vi "CollectISEOnly.vi"() -> ()   [LabVIEW 2016]
uses:
  <vilib>/Platform/TimedLoop/XDataNode/timing_clust.ctl
  <vilib>/Platform/TimedLoop/XDataNode/nitl_modes.ctl
  <vilib>/Platform/TimedLoop/XDataNode/wakeup.ctl
  <vilib>/Utility/file.llb/Write Delimited Spreadsheet (string).vi
  <vilib>/Platform/TimedLoop/XDataNode/loadnilvce.vi
  <vilib>/Utility/file.llb/Write Delimited Spreadsheet (DBL).vi
  <vilib>/Platform/TimedLoop/XDataNode/XDataNode.xnode
  <resource>/objmgr/ni.var.rc
  <vilib>/Platform/TimedLoop/XDataNode/XDNodeRunTimeDep.lvlib
panel:
  out "pH Live":dbl format="%#_4g"
  out "String 4":string="NH4"
  out "String 3":string="NH4"
  out "DO Live":dbl format="%#_4g"
  in  "Buffer Size":i32=100
  out "Saving?":bool
  out "new file path (Not A Path if cancelled)":path
  in  "File Name:":string
  out "Headers":string[](array[string])
  out "error out":errorcluster
  out "String 6":string="Na"
  out "NH4 Live":dbl format="%#_4g"
  out "Na Live":dbl format="%#_4g"
  out "current sample":dbl format="%#_3g"
  out "Date":string="K"
  out "Time":string="K"
  out "iter number":i32
  in  "stop":bool
  out "All data":dbl[][](array[numeric]) format="%#3.4f"
  in  "error in":errorcluster
  out "String 2":string="NH4"
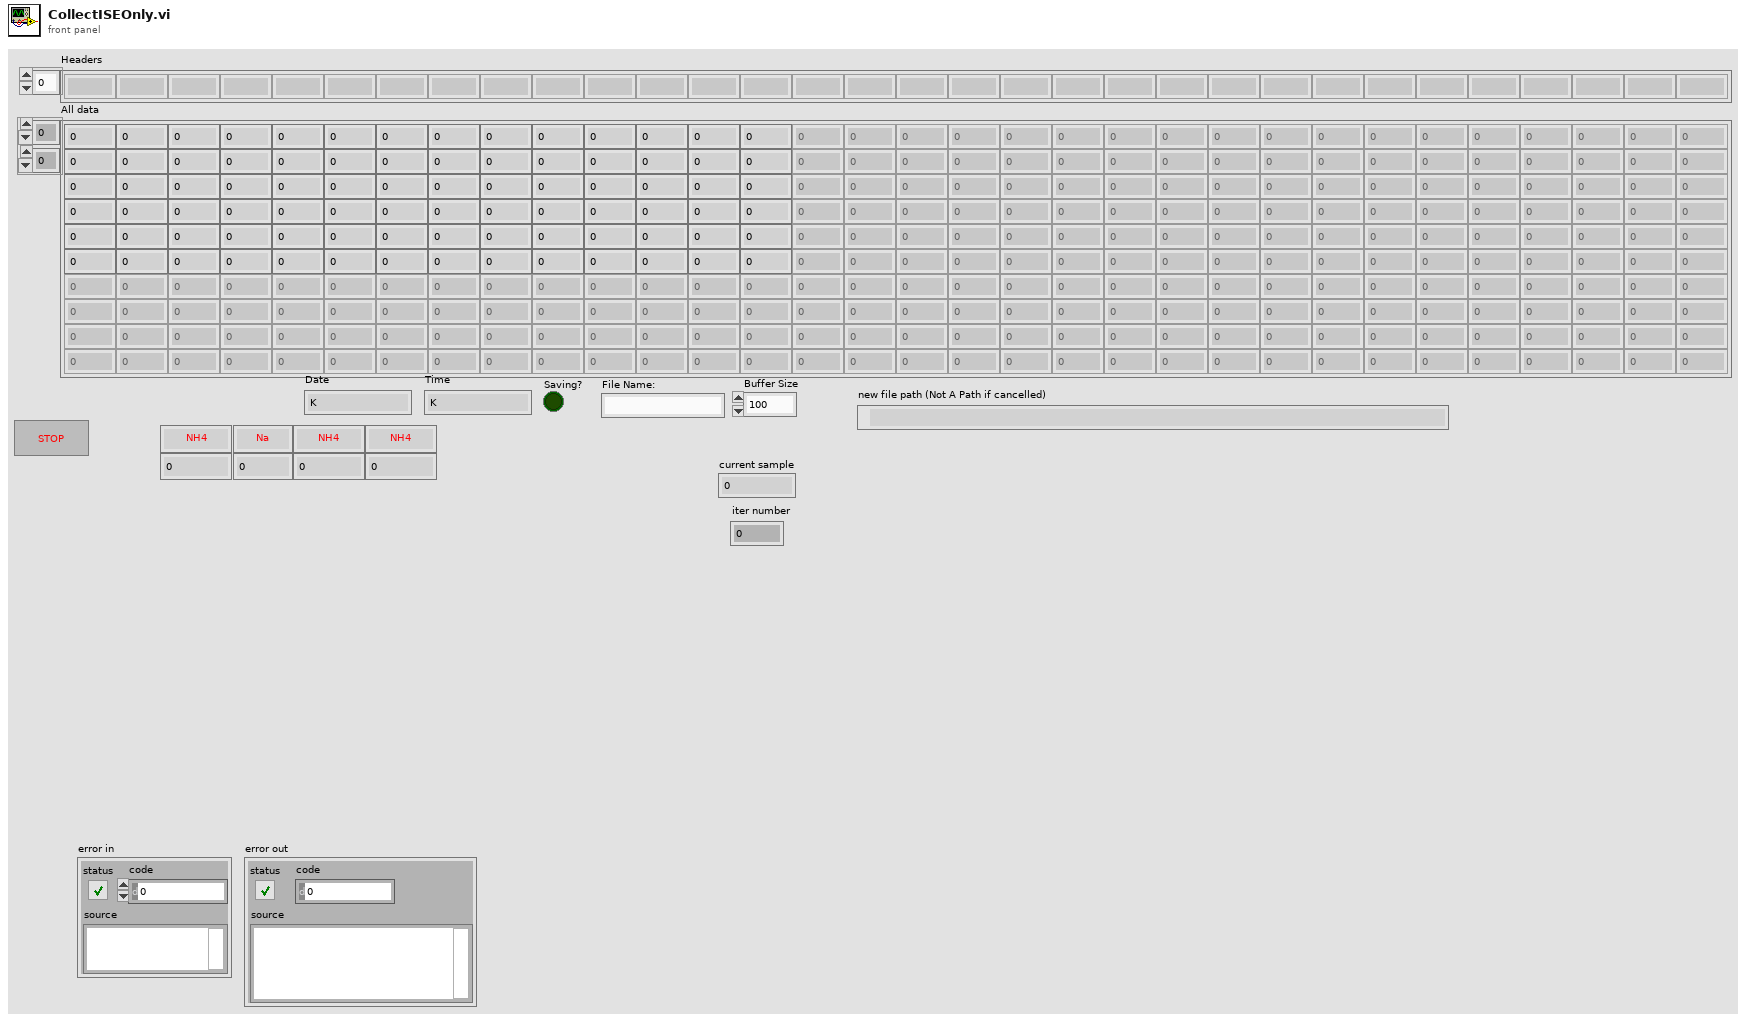
[diagram p1: front panel]
types:
  T1 = typedef "XDNodeRunTimeDep.lvlib/timing_clust.ctl" = cluster{"Expected End [f-1]":u64, "Actual End [f-1]":u64, "Finished Late? [f-1]":bool, "Expected End [i-1]":u64, "Actual End [i-1]":u64, "Finished Late? [i-1]":bool, "Expected Start [i]":u64, "Actual Start [i]":u64, "Expected Start [f]":u64, "Actual Start [f]":u64, "Source Name":string, "Structure Name":string, "Period":i64, "Deadline":i64, "Offset":i64, "Start":i64, "Priority":i32, "Timeout":i32, "Mode":T2, "Wakeup Reason":T3, "Error":errorcluster, "Source Type":string, "Secondary Source Type":string, "Global End Time":u64, "Global Start Time":u64, "Frame Duration":u64, "Iteration Duration":u64, "Assigned CPU":i32, "I/O Scan Engine Mode":u32}
  T2 = typedef "XDNodeRunTimeDep.lvlib/nitl_modes.ctl" = enum32{"No Change", "Process missed periods, maintain original phase", "Discard missed periods, maintain original phase", "Process missed periods, ignore original phase", "Discard missed periods, ignore original phase"}
  T3 = typedef "XDNodeRunTimeDep.lvlib/wakeup.ctl" = enum32{"Normal", "Aborted", "Asynchronous wakeup", "Timing source error", "Timed loop error", "Timeout"}
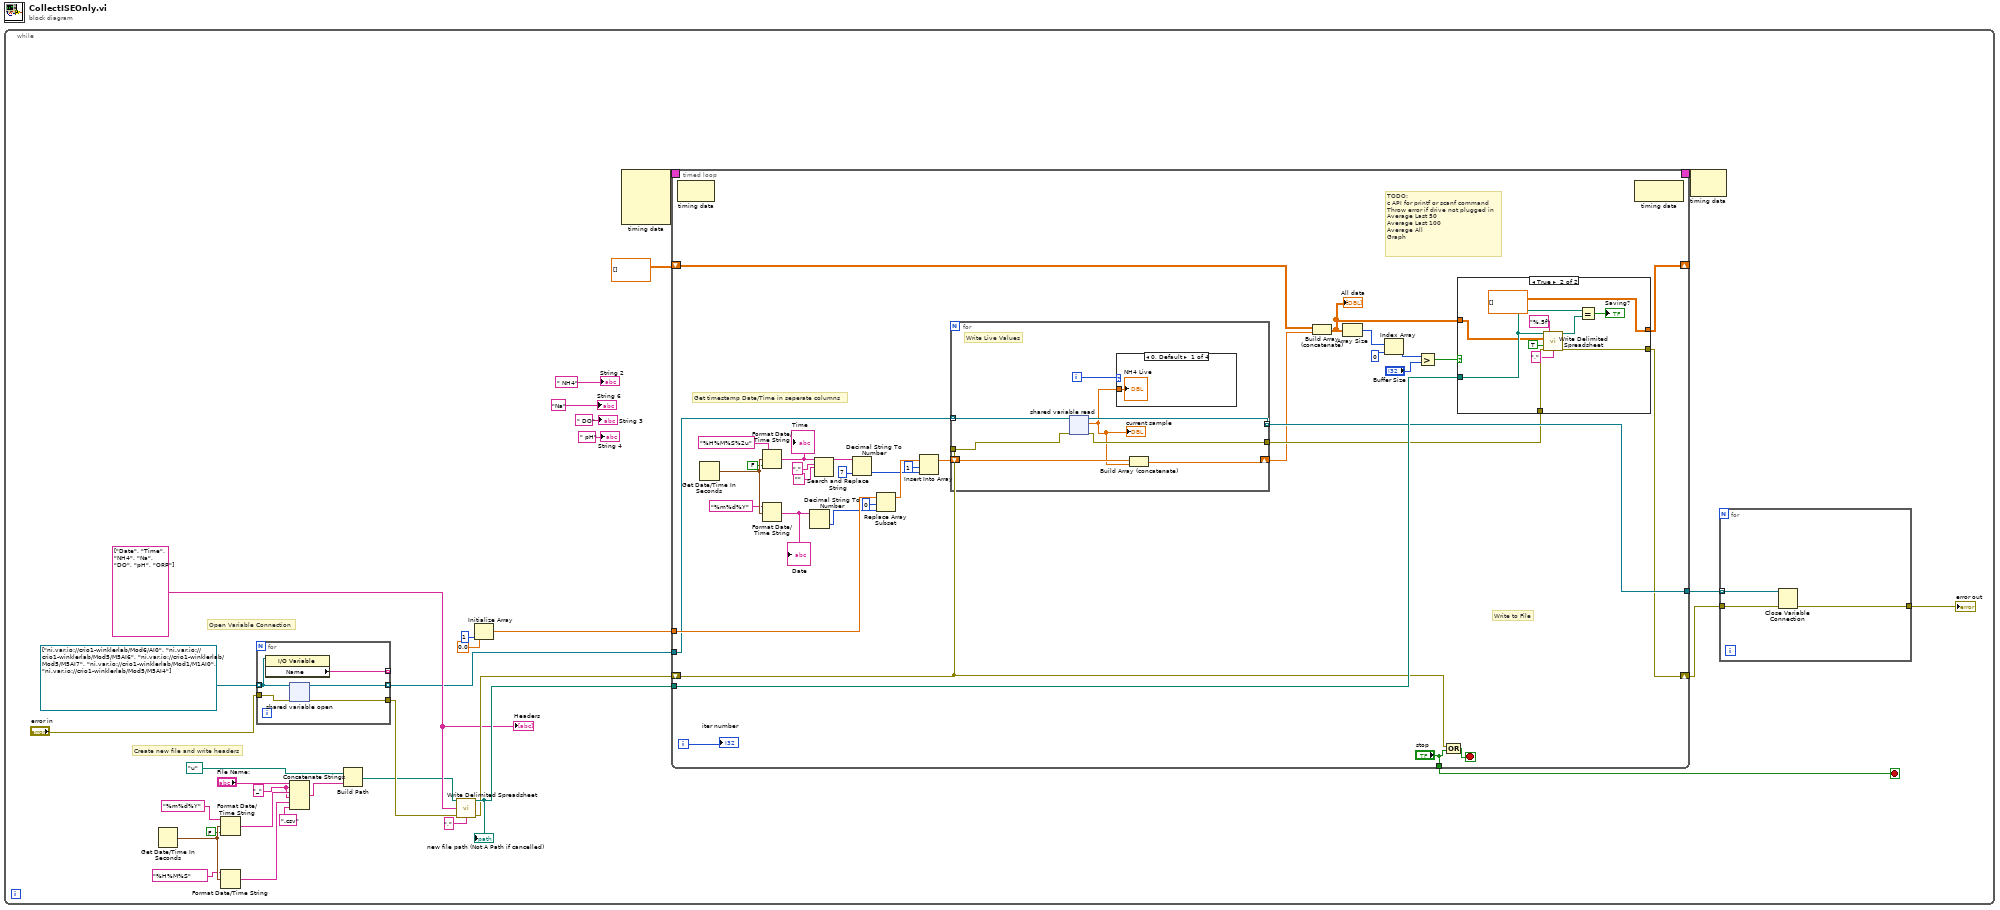
[diagram p0: block diagram]
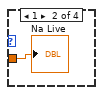
[diagram p3: hidden frame]
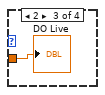
[diagram p4: hidden frame]
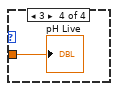
[diagram p5: hidden frame]
diagram:
  n1 = while {
    stop <- w6 stop-if-true
    w10 = "_" ("string")
    w25 = string[] ["Date", "Time", "NH4", "Na", "DO", "pH", "ORP"]
    # "Create new file and write headers"
    # "Open Variable Connection"
    n2 = Get Date/Time In Seconds() -> (seconds since 1Jan1904=w15:timestamp)
    n3 = Format Date/Time String(time format string (%c)="%m%d%Y", seconds (now)=w15, UTC format=FALSE) -> (date/time string=w11:string)
    n4 = Format Date/Time String(time format string (%c)="%H%M%S", seconds (now)=w15) -> (date/time string=w9:string)  [unwired: 1 in]
    n5 = for {
      tunnel: refnum<k21>[] ["ni.var.io://crio1-winklerlab/Mod6/AI0", "ni.var.io://crio1-winklerlab/Mod5/M5AI6", "ni.var.io://crio1-winklerlab/Mod5/M5AI7", "ni.var.io://crio1-winklerlab/Mod1/M1AI0", "ni.var.io://crio1-winklerlab/Mod5/M5AI4"] -> [w99] mode=indexing
      tunnel: "error in" -> [w102]
      tunnel: [w101] -> w22 mode=indexing
      tunnel: [w100] -> w20
      tunnel: [w98] -> _ mode=indexing
      n6 = property class="I/O Variable"(reference=w99) -> ("Name"=w98:string)  [unwired: 1 in, 2 out]
      n7 = shared-variable-open(w99, w102) -> (w101:refnum<k21>, w100:errorcluster)  [unwired: 1 in]
    }
    n8 = Concatenate Strings("File Name:", w10, w11, w10, w9, ".csv" ("string")) -> (w7:string)
    n9 = Build Path(base path=path "u:/" ("Save to:"), name or relative path=w7) -> (appended path=w19:path)
    n10 = call-poly <vilib>:"Write Delimited Spreadsheet.vi"("file path (dialog if empty)"=w19, "1D data"=w25, "error in (no error)"=w20, "delimiter (\\t)"="," ("delimiter (\\t)")) -> ("new file path (Not A Path if cancelled)"=w32:path, "error out"=w30:errorcluster)  [unwired: 10 in]
    "new file path (Not A Path if cancelled)" <- w32
    n11 = Initialize Array(0.0 ("element"), 1 ("dimension size")) -> (w33:dbl[])
    n12 = node-c288() -> (w5:T1)  [unwired: 4 in]
    n13 = timed-loop {
      tunnel: w33 -> [w60]
      tunnel: w32 -> [w46]
      shift-right: [w45] -> _
      shift-left: dbl[][] [] -> [w56]
      tunnel: w22 -> [w41]
      tunnel: [w43] -> w18
      shift-right: [w37] -> w8
      shift-left: w30 -> [w38]
      tunnel: ["stop"] -> w6
      timing: w5 -> [_]
      timing-out: [_] -> w4
      i -> [w57]
      stop <- w58 stop-if-true
      # "TODO: \nc API for printf or scanf command\nThrow error if drive not plugged in\nAverage Last 50\nAverage Last 100\nAverage All\nGraph"
      # "Write to File"
      # "Get timestamp Date/Time in seperate columns"
      n14 = node-c288() -> ()  [unwired: 1 in, 1 out]
      n15 = Get Date/Time In Seconds() -> (seconds since 1Jan1904=w68:timestamp)
      n16 = Format Date/Time String(time format string (%c)="%H%M%S%2u", seconds (now)=w68, UTC format=FALSE) -> (date/time string=w64:string)
      "Time" <- w64
      n17 = Format Date/Time String(time format string (%c)="%m%d%Y", seconds (now)=w68) -> (date/time string=w54:string)  [unwired: 1 in]
      "Date" <- w54
      n18 = Decimal String To Number(string=w54) -> (number=w53:i32)  [unwired: 2 in, 1 out]
      n19 = Search and Replace String(input string=w64, search string=".", replace string="") -> (result string=w63:string)  [unwired: 5 in, 3 out]
      n20 = Decimal String To Number(string=w63, default (0L)=7) -> (number=w52:i32)  [unwired: 1 in, 1 out]
      n21 = Replace Array Subset(array=w60, new element=w53, index=0) -> (w59:dbl[])
      n22 = Insert Into Array(array=w59, index=1, new element=w52) -> (w36:dbl[])
      n23 = for {
        tunnel: w38 -> [w91]
        shift-right: [w87] -> w40
        shift-left: w36 -> [w86]
        tunnel: [w90] -> w42
        tunnel: w41 -> [w89] mode=indexing
        tunnel: [w88] -> w43 mode=indexing
        i -> [w84]
        # "Write Live Values"
        n24 = shared-variable-read(w89, w91) -> (w88:refnum<k21>, w90:errorcluster, w85:dbl)  [unwired: 1 out]
        "current sample" <- w85
        n25 = case shown="0, Default" w84 {
          tunnel: w85 -> [w92 w93 w94 w95]
          frame 0, Default {
            "NH4 Live" <- w92
          }
          frame 1 {
            "Na Live" <- w93
          }
          frame 2 {
            "DO Live" <- w94
          }
          frame 3 {
            "pH Live" <- w95
          }
        }
        n26 = Build Array (concatenate)(w86, w85) -> (w87:dbl[])
      }
      n27 = Build Array (concatenate)(w56, w40) -> (w44:dbl[][])
      "All data" <- w44
      n28 = Array Size(array=w44) -> (size(s)=w50:i32[])
      n29 = Index Array(array=w50, index=0) -> (element=w48:i32)
      n30 = Greater?(x=w48, y="Buffer Size") -> (0:w47:bool)
      n31 = Compound Arithmetic op=OR(w38, "stop") -> (w58:bool)
      n32 = case shown="True" w47 {
        tunnel: w44 -> [w72 w80]
        tunnel: w46 -> [_ w81]
        tunnel: [w72 dbl[][] []] -> w45
        tunnel: w42 -> [w73 w79]
        tunnel: [w73 w78] -> w37
        frame False {
        }
        frame True {
          n33 = call-poly <vilib>:"Write Delimited Spreadsheet.vi"("file path (dialog if empty)"=w81, "format (%.3f)"="%.5f", "2D data"=w80, "append to file? (new file:F)"=TRUE, "error in (no error)"=w79, "delimiter (\\t)"="," ("delimiter (\\t)")) -> ("new file path (Not A Path if cancelled)"=w82:path, "error out"=w78:errorcluster)  [unwired: 8 in]
          n34 = Equal?(x=w81, y=w82) -> (x = y?=→"Saving?":bool)
        }
      }
      n35 = node-c288() -> ()  [unwired: 1 in, 1 out]
      "iter number" <- w57
    }
    n36 = node-c288(w4) -> ()  [unwired: 1 out]
    n37 = for {
      tunnel: [w105] -> w29
      tunnel: w18 -> [w104] mode=indexing
      tunnel: w8 -> [w103]
      n38 = Close Variable Connection(8:w103, 11:w104) -> (0:w105:errorcluster)
    }
    "error out" <- w29
    "String 2" <- " NH4"
    "String 6" <- "Na"
    "Headers" <- w25
    "String 3" <- " DO" ("String 3")
    "String 4" <- " pH" ("String 4")
  }
